vi "Get Resource Type.vi"(4 "UART in":refnum<class "UART.lvclass">) -> (7 "Resource Type":string)   [LabVIEW 2020, in "CTI.lvlib" / "UART.lvclass"]
uses:
  UART.lvclass
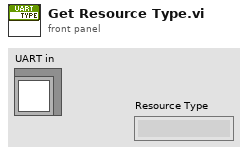
[diagram p1: front panel]
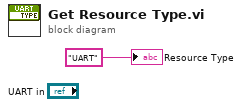
[diagram p0: block diagram]
diagram:
  "Resource Type" <- "UART" ("Resource Type")
